vi "5-3 VI run.vi"() -> ()   [LabVIEW 2014]
panel:
  out "에러 출력":errorcluster
  in  "vi 경로":path=path "C:/Users/LVEDU09/Documents/YSK/4-2 난수발생.vi"
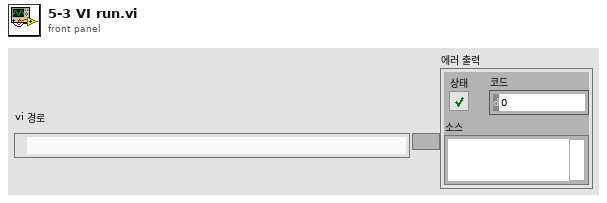
[diagram p1: front panel]
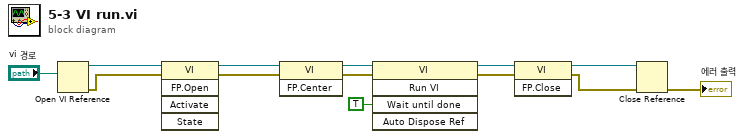
[diagram p0: block diagram]
diagram:
  n1 = Open VI Reference(vi path="vi 경로") -> (vi reference=w12:refnum<vi>, error out=w6:errorcluster)  [unwired: 5 in]
  n2 = invoke class="VI" method="FP.Open"(reference=w12, error in=w6) -> (reference out=w11:refnum<vi>, error out=w5:errorcluster)  [unwired: 3 in, 3 out]
  n3 = invoke class="VI" method="FP.Center"(reference=w11, error in=w5) -> (reference out=w10:refnum<vi>, error out=w4:errorcluster)  [unwired: 1 in, 1 out]
  n4 = invoke class="VI" method="Run VI"(reference=w10, error in=w4, "Wait until done"=TRUE ("완료될 때까지 기다림")) -> (reference out=w9:refnum<vi>, error out=w3:errorcluster)  [unwired: 2 in, 3 out]
  n5 = invoke class="VI" method="FP.Close"(reference=w9, error in=w3) -> (reference out=w8:refnum<vi>, error out=w2:errorcluster)  [unwired: 1 in, 1 out]
  n6 = Close Reference(reference=w8, error in (no error)=w2) -> (error out=→"에러 출력":errorcluster)
